vi "Prime BSI Capture.vi"(0 "Notifier In":refnum<notifier>, 7 "Camera Ref":refnum<k24>, 11 "Error In":errorcluster, 13 "Image Ref":T1) -> (4 "Notifier Out":refnum<notifier>, 8 "Prime Cluster":T2, 15 "Error Out":errorcluster)   [LabVIEW 2020]
uses:
  Prime BSI Type Defs/Prime BSI Notifier Element.ctl
  Prime BSI Type Defs/Prime BSI Actions.ctl
  Prime BSI Type Defs/Prime BSI Parameters.ctl
  Prime BSI Type Defs/Prime BSI Parameter List.ctl
  Prime BSI Type Defs/Prime BSI ROI.ctl
  <vilib>/vision/Image Controls.llb/IMAQ Image.ctl
  Camera Controls/Camera IMAQ Key Info.ctl
  Y:/Software/Photometrics/Photometrics LabView Package 2021/Dependencies/PVCamNET.dll
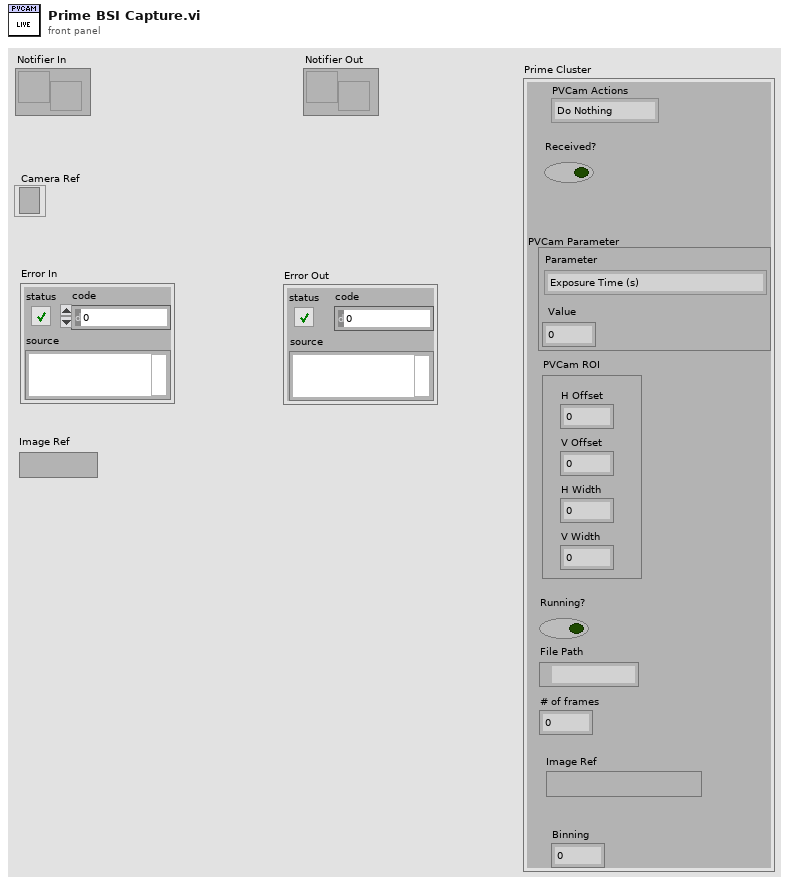
[diagram p1: front panel]
types:
  T1 = typedef "IMAQ Image.ctl" = refnum<image>
  T2 = typedef "Prime BSI Notifier Element.ctl" = cluster{"PVCam Actions":T3, "Received?":bool, "PVCam Parameter":T4, "PVCam ROI":T6, "Running?":bool, "File Path":path, "# of frames":u32, "Image Ref":T1, "Binning":i32}
  T3 = typedef "Prime BSI Actions.ctl" = enum16{"Do Nothing", "Preview", "Record", "Abort", "Record Settings", "Set Parameter", "Get Parameter", "Set ROI", "Get ROI", "Status", "Quit"}
  T4 = typedef "Prime BSI Parameters.ctl" = cluster{"Parameter":T5, "Value":dbl}
  T5 = typedef "Prime BSI Parameter List.ctl" = enum16{"Exposure Time (s)", "Binning"}
  T6 = typedef "Prime BSI ROI.ctl" = cluster{"H Offset":i32, "V Offset":i32, "H Width":i32, "V Width":i32}
  T7 = typedef "Camera IMAQ Key Info.ctl" = cluster{"Frame":u32, "Sensor Height":i32, "Sensor Width":i32, "ROI Height":i32, "ROI Width":i32, "ROI Enable?":bool, "Bit per Pixel":u8}
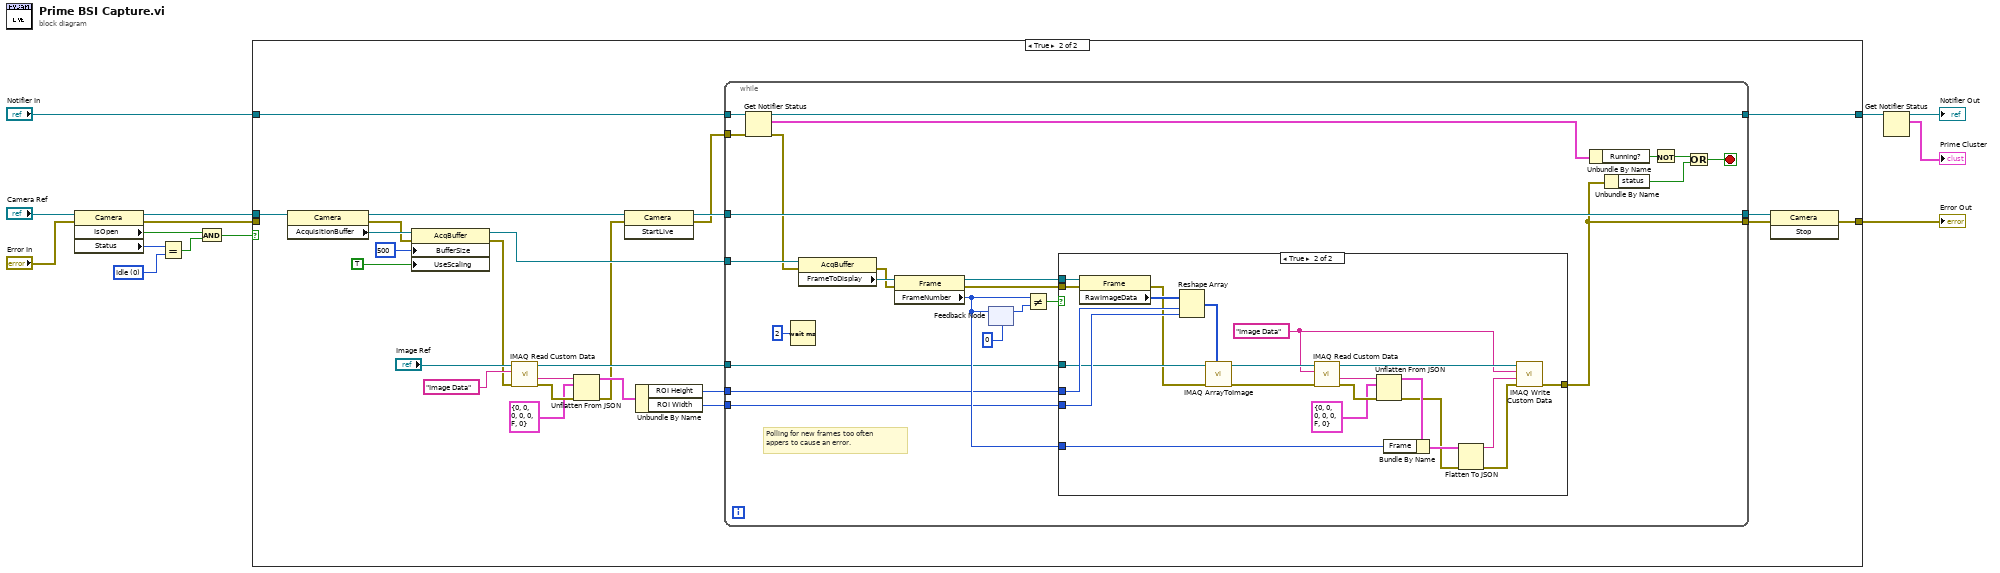
[diagram p0: block diagram]
diagram:
  w13 = 0 items=["Idle", "Capturing"] ("Status")
  n1 = property class="Camera"(reference="Camera Ref", error in="Error In") -> (reference out=w7:refnum<k24>, error out=w6:errorcluster, "IsOpen"=w12:bool, "Status"=w14:i32)
  n2 = Equal?(x=w14, y=w13) -> (x = y?=w11:bool)
  n3 = And(x=w12, y=w11) -> (x .and. y?=w8:bool)
  n4 = case shown="True" w8 {
    tunnel: w7 -> [_ w19]
    tunnel: w6 -> [w15 _]
    tunnel: "Notifier In" -> [w16 w38]
    tunnel: [w16 w34] -> w3
    tunnel: [w15 w33] -> w4
    frame False {
    }
    frame True {
      n5 = property class="Camera"(reference=w19) -> (reference out=w18:refnum<k24>, error out=w39:errorcluster, "AcquisitionBuffer"=w41:refnum<k24>)  [unwired: 1 in]
      n6 = property class="AcqBuffer"(reference=w41, error in=w39, "BufferSize"=u32 500, "UseScaling"=TRUE) -> (reference out=w32:refnum<k24>, error out=w25:errorcluster)
      n7 = call "IMAQ Read Custom Data"("error in (no error)"=w25, "Key"="Image Data", "Image"="Image Ref") -> ("error out"=w29:errorcluster, "Custom Data Out"=w30:string, "Image (duplicate)"=w22:T1)  [unwired: 6 in]
      n8 = Unflatten From JSON(JSON string=w30, type and defaults=T7 {"Frame"=0, "Sensor Height"=0, "Sensor Width"=0, "ROI Height"=0, "ROI Width"=0, "ROI Enable?"=FALSE, "Bit per Pixel"=0} ("Camera IMAQ Key Info"), error in (no error)=w29) -> (value=w26:T7, error out=w17:errorcluster)  [unwired: 4 in]
      n9 = invoke class="Camera" method="StartLive"(reference=w18, error in=w17) -> (reference out=w37:refnum<k24>, error out=w36:errorcluster)  [unwired: 1 in, 1 out]
      n10 = Unbundle By Name(w26) -> ("ROI Height"=w24:i32, "ROI Width"=w23:i32)
      n11 = while {
        tunnel: w38 -> [w65]
        tunnel: w37 -> [w57]
        tunnel: w36 -> [w63]
        tunnel: [w57] -> w35
        tunnel: [w58] -> w34
        tunnel: w32 -> [w56]
        tunnel: w24 -> [w48]
        tunnel: w23 -> [w47]
        tunnel: w22 -> [w49]
        tunnel: [w43] -> w21
        stop <- w61 stop-if-true
        # "Polling for new frames too often\nappers to cause an error."
        n12 = Get Notifier Status(notifier=w65, error in (no error)=w63) -> (notifier out=w58:refnum<notifier>, current notification=w59:T2, error out=w46:errorcluster)  [unwired: 2 out]
        n13 = Wait (ms)(milliseconds to wait=u32 2) -> ()  [unwired: 1 out]
        n14 = property class="AcqBuffer"(reference=w56, error in=w46) -> (error out=w45:errorcluster, "FrameToDisplay"=w55:refnum<k24>)  [unwired: 1 out]
        n15 = property class="Frame"(reference=w55, error in=w45) -> (reference out=w51:refnum<k24>, error out=w44:errorcluster, "FrameNumber"=w50:u32)
        n16 = feedback-in #1(w50) -> ()
        n17 = feedback #1(u32 0 ("FrameNumber")) -> (w53:u32)
        n18 = Not Equal?(x=w50, y=w53) -> (x != y?=w52:bool)
        n19 = case shown="True" w52 {
          tunnel: w51 -> [_ w88]
          tunnel: w50 -> [_ w77]
          tunnel: w49 -> [_ w84]
          tunnel: w48 -> [_ w86]
          tunnel: w47 -> [_ w85]
          tunnel: w44 -> [w66 w69]
          tunnel: [w66 w67] -> w43
          frame False {
          }
          frame True {
            w70 = "Image Data" ("Key")
            n20 = property class="Frame"(reference=w88, error in=w69) -> (error out=w68:errorcluster, "RawImageData"=w87:u16[])  [unwired: 1 out]
            n21 = Reshape Array(w87, w86, w85) -> (w83:u16[][])
            n22 = call "IMAQ ArrayToImage"("Image Pixels (U16)"=w83, "error in (no error)"=w68, "Image"=w84) -> ("error out"=w78:errorcluster, "Image Out"=w79:T1)  [unwired: 7 in]
            n23 = call "IMAQ Read Custom Data"("error in (no error)"=w78, "Key"=w70, "Image"=w79) -> ("error out"=w81:errorcluster, "Custom Data Out"=w82:string, "Image (duplicate)"=w75:T1)  [unwired: 6 in]
            n24 = Unflatten From JSON(JSON string=w82, type and defaults=T7 {"Frame"=0, "Sensor Height"=0, "Sensor Width"=0, "ROI Height"=0, "ROI Width"=0, "ROI Enable?"=FALSE, "Bit per Pixel"=0} ("Camera IMAQ Key Info"), error in (no error)=w81) -> (value=w76:T7, error out=w73:errorcluster)  [unwired: 4 in]
            n25 = Bundle By Name(cluster=w76, "Frame"=w77) -> (w74:T7)
            n26 = Flatten To JSON(anything=w74, error in (no error)=w73) -> (JSON string=w72:string, 11:w71:errorcluster)  [unwired: 1 in]
            n27 = call "IMAQ Write Custom Data"("error in (no error)"=w71, "Custom Data In"=w72, "Key"=w70, "Image"=w75) -> ("error out"=w67:errorcluster)  [unwired: 6 in, 1 out]
          }
        }
        n28 = Unbundle By Name(w59) -> ("Running?"=w64:bool)
        n29 = Unbundle By Name(w43) -> ("status"=w60:bool)
        n30 = Not(x=w64) -> (.not. x?=w62:bool)
        n31 = Or(x=w62, y=w60) -> (x .or. y?=w61:bool)
      }
      n32 = invoke class="Camera" method="Stop"(reference=w35, error in=w21) -> (error out=w33:errorcluster)  [unwired: 1 in, 2 out]
    }
  }
  "Error Out" <- w4
  n33 = Get Notifier Status(notifier=w3) -> (notifier out=→"Notifier Out":refnum<notifier>, current notification=→"Prime Cluster":T2)  [unwired: 1 in, 3 out]
